vi "GetParam.vi"(8 "error in (no error)":errorcluster caption="entrée d'erreur (pas d'erreur)", 11 "Biclusters.lvclass":refnum<class "Biclusters.lvclass">) -> (0 "error out":errorcluster caption="sortie d'erreur", 2 "make_biclusters":T1={"n_rows"=300, "n_cols"=300, "n_clusters"=5, "noise"=5.0, "minval"=10, "maxval"=100, "shuffle"=TRUE, "random_state"=-1, "Returns"="X"} {"random_state" min=-1; "n_clusters" min=1; "n_cols" min=1; "n_rows" min=1}, 3 "Biclusters.lvclass":refnum<class "Biclusters.lvclass">)   [LabVIEW 2020, in "Biclusters.lvclass"]
doc: "Get Parameters"
uses:
  Biclusters.lvclass
  Biclusters.lvclass/Biclusters.ctl
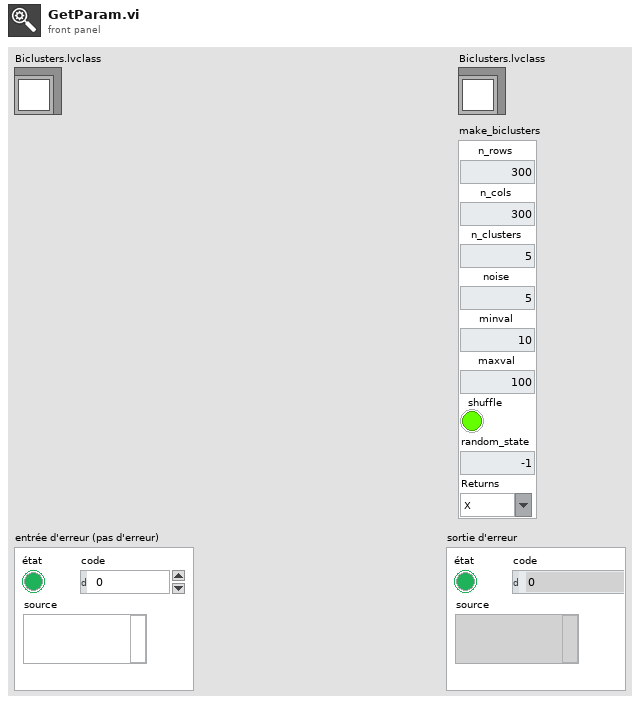
[diagram p1: front panel]
types:
  T1 = cluster{"n_rows":u32, "n_cols":u32, "n_clusters":u32, "noise":dbl, "minval":i32, "maxval":i32, "shuffle":bool, "random_state":i32, "Returns":string}
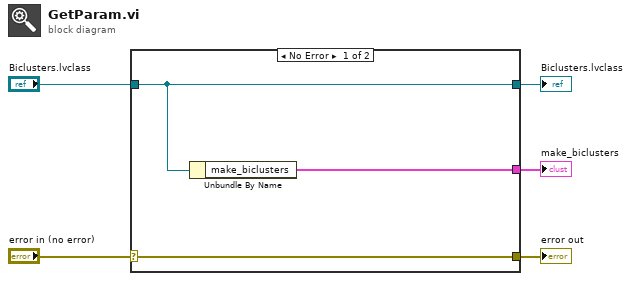
[diagram p0: block diagram]
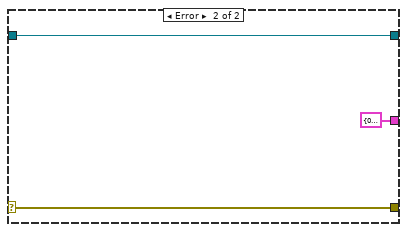
[diagram p2: hidden frame]
diagram:
  n1 = case shown="No Error" "error in (no error)" {
    selector: "error in (no error)" -> [w8 w10]
    tunnel: [w8 w10] -> w4
    tunnel: [w7 w11] -> w2
    tunnel: "Biclusters.lvclass" -> [w7 w11]
    tunnel: [w6 T1 {"n_rows"=0, "n_cols"=0, "n_clusters"=0, "noise"=0.0, "minval"=0, "maxval"=0, "shuffle"=FALSE, "random_state"=0, "Returns"=""} ("make_biclusters")] -> w1
    frame No Error {
      n2 = Unbundle By Name(w7) -> ("make_biclusters"=w6:T1)
    }
    frame Error {
    }
  }
  "error out" <- w4
  "Biclusters.lvclass" <- w2
  "make_biclusters" <- w1
